vi "Remove_Escaped_Char.vi"(1 "Offset":i32, 2 "Input String":string) -> (0 "Output String":string)   [LabVIEW 2011]
doc: "This VI returns the character in a string at the given offset, unless that character was escaped with a backslash, in which case it returns nothing."
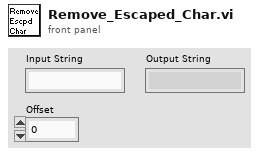
[diagram p1: front panel]
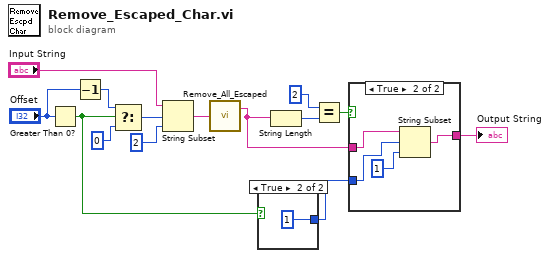
[diagram p0: block diagram]
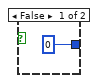
[diagram p2: hidden frame]
diagram:
  n1 = Greater Than 0?(x="Offset") -> (x > 0?=w4:bool)
  n2 = Decrement(x="Offset") -> (x-1=w13:i32)
  n3 = Select(t=w13, s=w4, f=u32 0 ("Position")) -> (s? t:f=w12:u32)
  n4 = String Subset(string="Input String", offset (0)=w12, length (rest)=2 ("length (rest)")) -> (substring=w2:string)
  n5 = call "Remove_All_Escaped.vi"("Input String"=w2) -> ("Output String"=w1:string)  [unwired: 1 out]
  n6 = case shown="True" w4 {
    tunnel: [0 ("offset (0)") 1 ("offset (0)")] -> w3
    frame False {
    }
    frame True {
    }
  }
  n7 = String Length(string=w1) -> (length=w10:i32)
  n8 = Equal?(x=2, y=w10) -> (x = y?=w7:bool)
  n9 = case shown="True" w7 {
    tunnel: w1 -> [w17 w21]
    tunnel: [w17 w20] -> w8
    tunnel: w3 -> [_ w18]
    frame False {
    }
    frame True {
      n10 = String Subset(string=w21, offset (0)=w18, length (rest)=1 ("length (rest)")) -> (substring=w20:string)
    }
  }
  "Output String" <- w8
